vi "Tacking Helper - Tack Plotter.vi"(11 "Intermediate\nWaypoints In":T1[](array[typedef]) {"UTM Location"."North" format="%#_10f"; "UTM Location"."East" format="%#_8f"}) -> (3 "Tack Plot Data Out":cluster{dbl[], dbl[]}[](array[cluster]))   [LabVIEW 2011]
doc: "The for loop scans through the tack points and packages them for plotting - separate arrays for x and y data clustered together for plotting in the front panel.\n\nThe initialized array at the end of the vi creates an array of the clusters, so that multiple plots can be plotted at once - the wind plot element is currently added to this array in the main vi"
uses:
  2 Typedefs/UTM Location.ctl
  0x2-OCU-Think Comm/0x2 Typedefs/ocuWaypoint.ctl
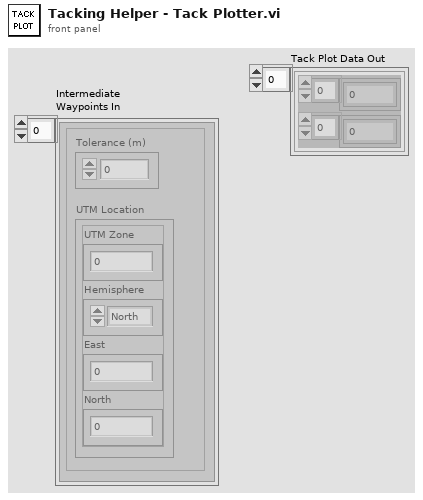
[diagram p1: front panel]
types:
  T1 = typedef "ocuWaypoint.ctl" = cluster{"Tolerance (m)":dbl, "UTM Location":T2}
  T2 = typedef "UTM Location.ctl" = cluster{"UTM Zone":dbl, "Hemisphere":enum16{"North", "South"}, "East":dbl, "North":dbl}
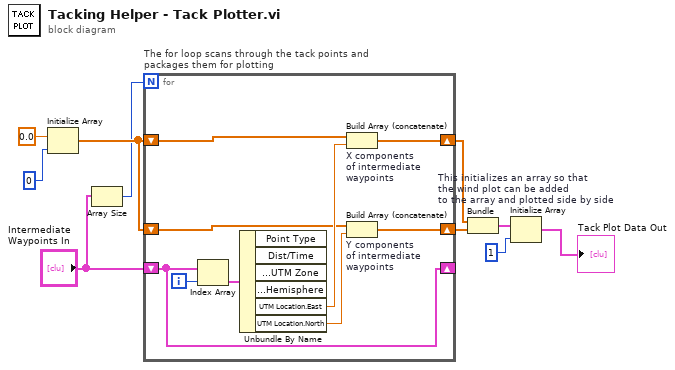
[diagram p0: block diagram]
diagram:
  n1 = Initialize Array "Initialize Array"(0.0 ("element"), 0 ("dimension size")) -> (w7:dbl[])
  n2 = Array Size(array="Intermediate\nWaypoints In") -> (size(s)=w1:i32)
  n3 = for "The for loop scans through the tack points and\npackages them for plotting" {
    N: w1 -> [_]
    shift-right: [w18] -> _
    shift-left: "Intermediate\nWaypoints In" -> [w18]
    shift-right: [w15] -> w5
    shift-left: w7 -> [w14]
    shift-right: [w11] -> w6
    shift-left: w7 -> [w13]
    i -> [w17]
    n4 = Index Array(array=w18, index=w17) -> (element=w19:T1)
    n5 = Unbundle By Name(w19) -> ("UTM Location.East"=w16:dbl, "UTM Location.North"=w12:dbl)  [unwired: 4 out]
    n6 = Build Array (concatenate) "X components\nof intermediate\nwaypoints"(w14, w16) -> (w15:dbl[])
    n7 = Build Array (concatenate) "Y components\nof intermediate\nwaypoints"(w13, w12) -> (w11:dbl[])
  }
  n8 = Bundle(w5, w6) -> (w8:cluster{dbl[], dbl[]})  [unwired: 1 in]
  n9 = Initialize Array "This initializes an array so that\nthe wind plot can be added\nto the array and plotted side by side"(w8, 1 ("dimension size")) -> (→"Tack Plot Data Out":cluster{dbl[], dbl[]}[])
